vi "LINE.vi"(0 "FG Voltage(mV)":dbl, 1 "Laser GPIB":u8=10 max=100, 2 "Mode":bool=TRUE, 3 "VISA resource name":refnum<visa-resource-name>="COM5", 4 "y-dist":i32, 5 "x-dist":i32, 6 "speed":u16, 7 "Motor GPIB":u8=6) -> ()   [LabVIEW 2012]
doc: "Mode:\nTrue - Write a striaght where Arduino is triggered using this program \"LINE.vi\"\nFalse - Write a striaght where Arduino is triggered externally (by other program)"
uses:
  <vilib>/Instr/_visa.llb/VISA Configure Serial Port (Instr).vi
  <vilib>/express/express arith-compare/Formula/XNode/ExpressFormulaBlockNode.xnode
panel:
  in  "Current (mA)":dbl=2.0
  in  "FG GPIB":u8=1
  in  "turn off delay (ms)":u16=55
  in  "turn on delay (ms)":u16=55
  # "LINE<space>[Displacement]<space>[Speed]<space>[voltage]"
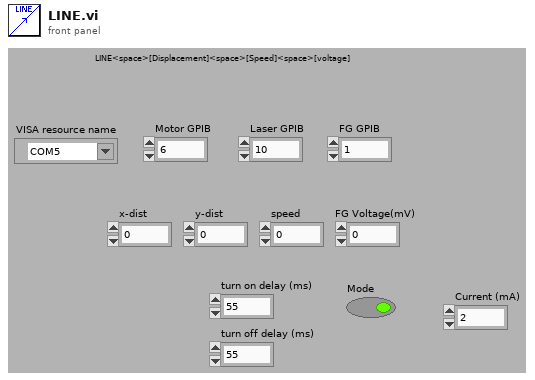
[diagram p1: front panel]
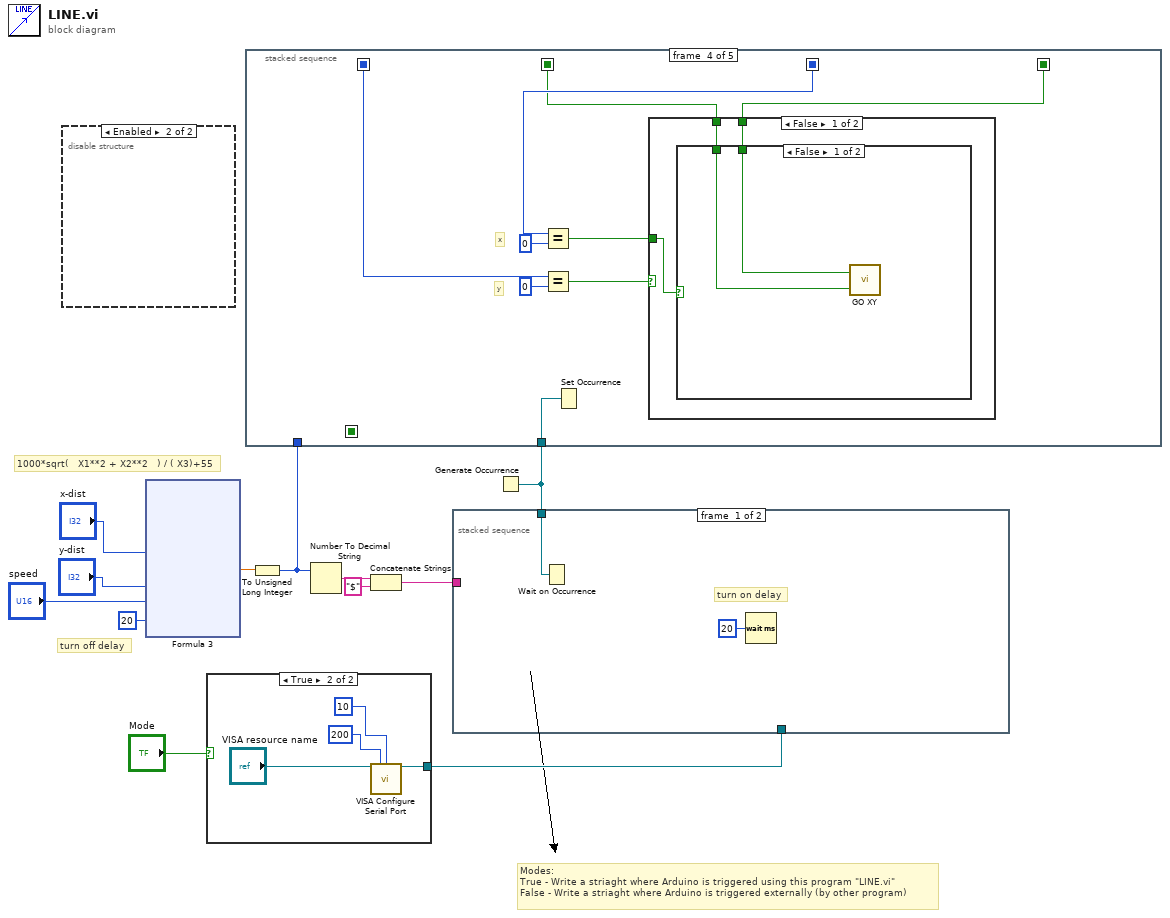
[diagram p0: block diagram]
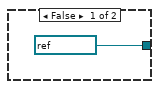
[diagram p2: hidden frame]
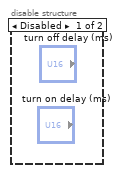
[diagram p3: hidden frame]
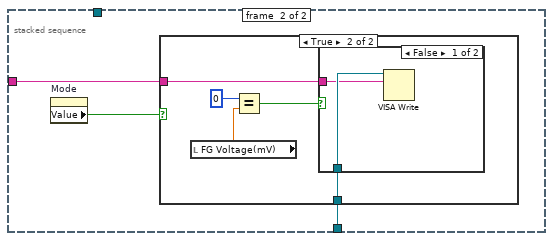
[diagram p4: hidden frame]
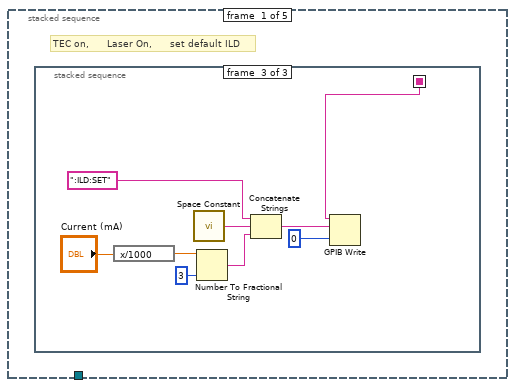
[diagram p7: hidden frame]
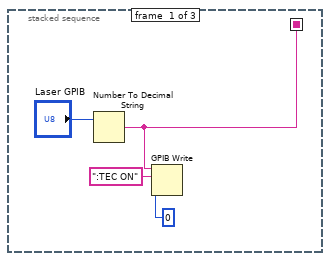
[diagram p8: hidden frame]
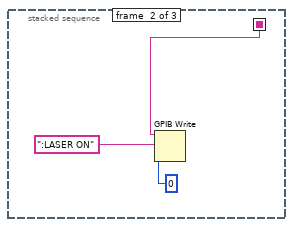
[diagram p9: hidden frame]
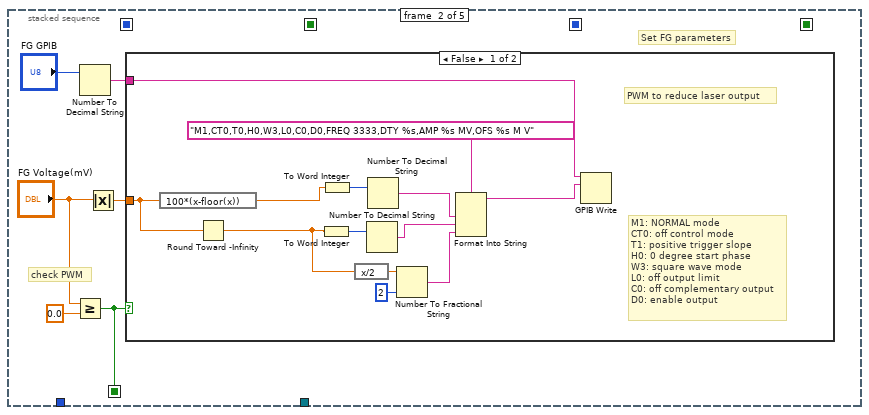
[diagram p10: hidden frame]
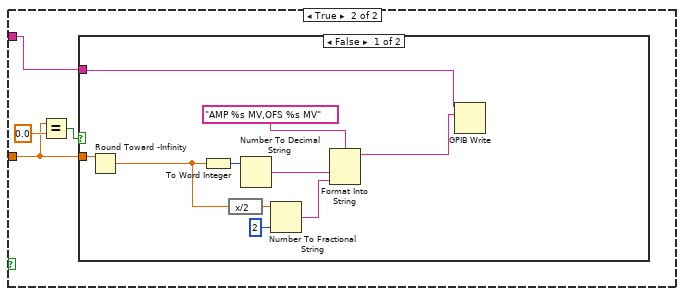
[diagram p11: hidden frame]
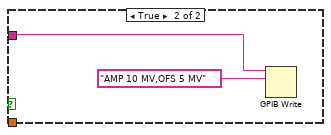
[diagram p12: hidden frame]
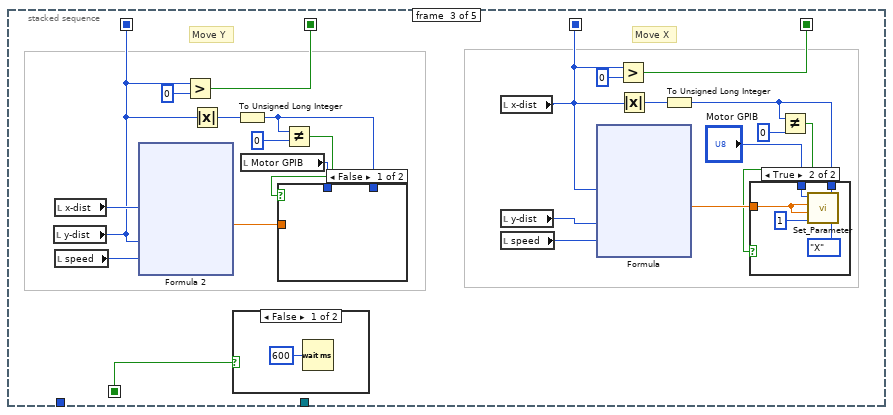
[diagram p13: hidden frame]
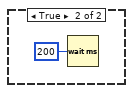
[diagram p14: hidden frame]
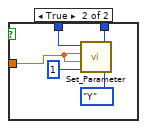
[diagram p16: hidden frame]
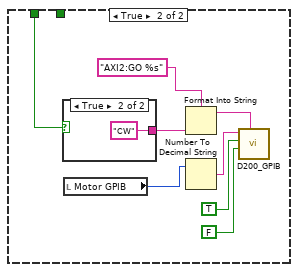
[diagram p17: hidden frame]
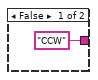
[diagram p18: hidden frame]
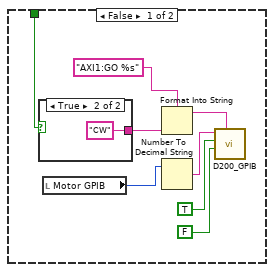
[diagram p20: hidden frame]
diagram:
  # "turn off delay"
  # "Modes:\nTrue - Write a striaght where Arduino is triggered using this program \"LINE.vi\"\nFalse - Write a striaght where Arduino is triggered externally (by other program)"
  # "1000*sqrt(   X1**2 + X2**2   ) / ( X3)+55"
  n1 = disable-structure shown="Enabled" {
    frame Disabled {
    }
    frame Enabled {
    }
  }
  n2 = xnode "Formula 3"("X1"="x-dist", "X2"="y-dist", "X3"="speed", "X4"=u16 20) -> ("Result"=w3:dbl)  [unwired: 1 in, 1 out]
  n3 = case shown="True" "Mode" {
    tunnel: [refnum<visa-resource-name> "COM5" ("VISA resource name out") w14] -> w10
    frame False {
    }
    frame True {
      n4 = call-poly "VISA Configure Serial Port"("VISA resource name"="VISA resource name", "timeout (10sec)"=u32 200, "termination char\n(0xA = '\\n' = LF)"=u8 10 ("termination char\n(0xA = '\\n' = LF)")) -> ("VISA resource name out"=w14:refnum<visa-resource-name>)  [unwired: 11 in, 1 out]
    }
  }
  n5 = To Unsigned Long Integer(number=w3) -> (unsigned 32bit integer=w2:u32)
  n6 = Number To Decimal String(number=w2) -> (decimal integer string=w6:string)  [unwired: 1 in]
  n7 = Concatenate Strings(w6, "$" ("string")) -> (w5:string)
  n8 = Generate Occurrence() -> (w12:refnum<k4>)
  n9 = stacked-sequence {
    seq-local: [_ _ w75 _ _] -> [_ _ _ w129 _]
    seq-local: [_ _ w74 _ _] -> [_ _ _ w130 _]
    seq-local: [_ _ w73 _ _] -> [_ _ _ w136 _]
    seq-local: [_ _ w72 _ _] -> [_ _ _ w134 _]
    seq-local: [_ w34 _ _ _] -> [_ _ w69 _ _]
    tunnel: w12 -> [_ _ _ w128 _]
    tunnel: w2 -> [_ _ _ _ w164]
    frame #0 {
      # "TEC on,      Laser On,      set default ILD"
      n10 = stacked-sequence {
        seq-local: [w18 _ _] -> [_ w22 w32]
        frame #0 {
          n11 = Number To Decimal String(number="Laser GPIB") -> (decimal integer string=w18:string)  [unwired: 1 in]
          n12 = GPIB Write(0:w18, 1:":TEC ON" ("data"), 2:i16 0 ("mode (0)")) -> ()  [unwired: 2 in, 2 out]
        }
        frame #1 {
          n13 = GPIB Write(0:w22, 1:":LASER ON" ("data"), 2:i16 0 ("mode (0)")) -> ()  [unwired: 2 in, 2 out]
        }
        frame #2 {
          n14 = expression code="x/1000"("Current (mA)") -> (w31:dbl)
          n15 = call <vilib>:"Space Constant.vi"() -> ("String"=w26:string)
          n16 = Number To Fractional String(number=w31, precision (6)=i16 3) -> (F-format string=w28:string)  [unwired: 2 in]
          n17 = Concatenate Strings(":ILD:SET", w26, w28) -> (w25:string)
          n18 = GPIB Write(0:w32, 1:w25, 2:i16 0 ("mode (0)")) -> ()  [unwired: 2 in, 2 out]
        }
      }
    }
    frame #1 {
      # "check PWM"
      # "Set FG parameters"
      n19 = Greater Or Equal?(x="FG Voltage(mV)", y=0.0) -> (x >= y?=w34:bool)
      n20 = Number To Decimal String(number="FG GPIB") -> (decimal integer string=w37:string)  [unwired: 1 in]
      n21 = Absolute Value(x="FG Voltage(mV)") -> (abs(x)=w35:dbl)
      n22 = case shown="False" w34 {
        tunnel: w37 -> [w49 w53]
        tunnel: w35 -> [w43 w55]
        frame False {
          # "PWM to reduce laser output"
          # "M1: NORMAL mode\nCT0: off control mode\nT1: positive trigger slope\nH0: 0 degree start phase\nW3: square wave mode\nL0: off output limit\nC0: off complementary output\nD0: enable output"
          n23 = expression code="100*(x-floor(x))"(w43) -> (w41:dbl)
          n24 = Round Toward -Infinity(1:w43) -> (0:w47:dbl)
          n25 = To Word Integer(number=w47) -> (16bit integer=w48:i16)
          n26 = To Word Integer(number=w41) -> (16bit integer=w42:i16)
          n27 = expression code="x/2"(w47) -> (w52:dbl)
          n28 = Number To Decimal String(number=w48) -> (decimal integer string=w44:string)  [unwired: 1 in]
          n29 = Number To Decimal String(number=w42) -> (decimal integer string=w40:string)  [unwired: 1 in]
          n30 = Number To Fractional String(number=w52, precision (6)=i16 2) -> (F-format string=w45:string)  [unwired: 2 in]
          n31 = Format Into String(format string="M1,CT0,T0,H0,W3,L0,C0,D0,FREQ 3333,DTY %s,AMP %s MV,OFS %s M V", w40, w44, w45) -> (resulting string=w50:string)  [unwired: 2 in, 1 out]
          n32 = GPIB Write(0:w49, 1:w50) -> ()  [unwired: 3 in, 2 out]
        }
        frame True {
          n33 = Equal?(x=w55, y=0.0) -> (x = y?=w54:bool)
          n34 = case shown="False" w54 {
            tunnel: w53 -> [w59 w68]
            tunnel: w55 -> [w57 _]
            frame False {
              n35 = Round Toward -Infinity(1:w57) -> (0:w58:dbl)
              n36 = To Word Integer(number=w58) -> (16bit integer=w60:i16)
              n37 = expression code="x/2"(w58) -> (w65:dbl)
              n38 = Number To Decimal String(number=w60) -> (decimal integer string=w62:string)  [unwired: 1 in]
              n39 = Number To Fractional String(number=w65, precision (6)=i16 2) -> (F-format string=w66:string)  [unwired: 2 in]
              n40 = Format Into String(format string="AMP %s MV,OFS %s MV", w62, w66) -> (resulting string=w61:string)  [unwired: 2 in, 1 out]
              n41 = GPIB Write(0:w59, 1:w61) -> ()  [unwired: 3 in, 2 out]
            }
            frame True {
              n42 = GPIB Write(0:w68, 1:"AMP 10 MV,OFS 5 MV") -> ()  [unwired: 3 in, 2 out]
            }
          }
        }
      }
    }
    frame #2 {
      # "Move X"
      # "Move Y"
      n43 = local read "y-dist"() -> (w73:i32)
      n44 = local read "x-dist"() -> (w88:i32)
      n45 = local read "speed"() -> (w91:u16)
      n46 = xnode "Formula 2"("X1"=w88, "X2"=w73, "X3"=w91) -> ("Result"=w83:dbl)  [unwired: 1 in, 1 out]
      n47 = Greater?(x=w73, y=0) -> (0:w75:bool)
      n48 = Absolute Value(x=w73) -> (abs(x)=w87:i32)
      n49 = case shown="False" w69 {
        frame False {
          n50 = Wait (ms)(milliseconds to wait=u32 600) -> ()  [unwired: 1 out]
        }
        frame True {
          n51 = Wait (ms)(milliseconds to wait=u32 200) -> ()  [unwired: 1 out]
        }
      }
      n52 = To Unsigned Long Integer(number=w87) -> (unsigned 32bit integer=w81:u32)
      n53 = local read "Motor GPIB"() -> (w90:u8)
      n54 = Not Equal?(x=w81, y=u32 0) -> (x != y?=w79:bool)
      n55 = case shown="False" w79 {
        tunnel: w90 -> [_ w101]
        tunnel: w81 -> [_ w100]
        tunnel: w83 -> [_ w99]
        frame False {
        }
        frame True {
          n56 = call "Set_Parameter.vi"("Axis"=enum16{"X", "Y", "Z", "U", "V", "W"}."Y", "Distance"=w100, "Rate"=u16 1, "L Speed"=w99, "F Speed"=w99, "GPIB_Addr"=w101) -> ()
        }
      }
      n57 = local read "x-dist"() -> (w72:i32)
      n58 = local read "y-dist"() -> (w71:i32)
      n59 = local read "speed"() -> (w70:u16)
      n60 = xnode "Formula"("X1"=w72, "X2"=w71, "X3"=w70) -> ("Result"=w82:dbl)  [unwired: 1 in, 1 out]
      n61 = Greater?(x=w72, y=0) -> (0:w74:bool)
      n62 = Absolute Value(x=w72) -> (abs(x)=w84:i32)
      n63 = To Unsigned Long Integer(number=w84) -> (unsigned 32bit integer=w78:u32)
      n64 = Not Equal?(x=w78, y=u32 0) -> (x != y?=w76:bool)
      n65 = case shown="True" w76 {
        tunnel: "Motor GPIB" -> [_ w98]
        tunnel: w78 -> [_ w95]
        tunnel: w82 -> [_ w94]
        frame False {
        }
        frame True {
          n66 = call "Set_Parameter.vi"("Axis"=enum16{"X", "Y", "Z", "U", "V", "W"}."X", "Distance"=w95, "Rate"=u16 1, "L Speed"=w94, "F Speed"=w94, "GPIB_Addr"=w98) -> ()
        }
      }
    }
    frame #3 {
      # "x"
      # "y"
      n67 = Equal?(x=w134, y=0) -> (x = y?=w132:bool)
      n68 = Equal?(x=w136, y=0) -> (x = y?=w131:bool)
      n69 = Set Occurrence(w128) -> ()
      n70 = case shown="False" w131 {
        tunnel: w132 -> [w138 w153]
        tunnel: w130 -> [w137 w152]
        tunnel: w129 -> [w139 _]
        frame False {
          n71 = case shown="False" w138 {
            tunnel: w139 -> [w141 w143]
            tunnel: w137 -> [w140 _]
            frame False {
              n72 = call "GO XY.vi"("Y-axis"=w141, "X-axis"=w140) -> ()  [unwired: 1 in]
            }
            frame True {
              n73 = case shown="True" w143 {
                tunnel: ["CCW" "CW"] -> w148
                frame False {
                }
                frame True {
                }
              }
              n74 = local read "Motor GPIB"() -> (w142:u8)
              n75 = Format Into String(format string="AXI2:GO %s", w148) -> (resulting string=w145:string)  [unwired: 2 in, 1 out]
              n76 = Number To Decimal String(number=w142) -> (decimal integer string=w144:string)  [unwired: 1 in]
              n77 = call "D200_GPIB.vi"("GPIB\nAddress"=w144, "Write"=TRUE, "Read"=FALSE, "Characters to Write"=w145) -> ()  [unwired: 1 in, 3 out]
            }
          }
        }
        frame True {
          n78 = case shown="True" w153 {
            tunnel: w152 -> [w155 _]
            frame False {
              n79 = case shown="True" w155 {
                tunnel: ["CCW" "CW"] -> w160
                frame False {
                }
                frame True {
                }
              }
              n80 = local read "Motor GPIB"() -> (w154:u8)
              n81 = Format Into String(format string="AXI1:GO %s", w160) -> (resulting string=w157:string)  [unwired: 2 in, 1 out]
              n82 = Number To Decimal String(number=w154) -> (decimal integer string=w156:string)  [unwired: 1 in]
              n83 = call "D200_GPIB.vi"("GPIB\nAddress"=w156, "Write"=TRUE, "Read"=FALSE, "Characters to Write"=w157) -> ()  [unwired: 1 in, 3 out]
            }
            frame True {
            }
          }
        }
      }
    }
    frame #4 {
      n84 = Wait (ms)(milliseconds to wait=w164) -> ()  [unwired: 1 out]
    }
  }
  n85 = stacked-sequence {
    tunnel: w12 -> [w166 _]
    tunnel: w10 -> [_ w169]
    tunnel: w5 -> [_ w168]
    frame #0 {
      # "turn on delay"
      n86 = Wait on Occurrence(2:w166) -> ()  [unwired: 2 in, 1 out]
      n87 = Wait (ms)(milliseconds to wait=u32 20) -> ()  [unwired: 1 out]
    }
    frame #1 {
      n88 = property on="Mode" class="Bool (strict)"() -> ("Value"=w167:bool)  [unwired: 2 in, 2 out]
      n89 = case shown="True" w167 {
        tunnel: w169 -> [_ w171]
        tunnel: w168 -> [_ w170]
        frame False {
        }
        frame True {
          n90 = local read "FG Voltage(mV)"() -> (w174:dbl)
          n91 = Equal?(x=0, y=w174) -> (x = y?=w172:bool)
          n92 = case shown="False" w172 {
            tunnel: w171 -> [w176 _]
            tunnel: w170 -> [w175 _]
            frame False {
              n93 = VISA Write(VISA resource name=w176, write buffer=w175) -> ()  [unwired: 1 in, 3 out]
            }
            frame True {
            }
          }
        }
      }
    }
  }
